vi "register_voltage.vi"(8 "error in (no error)":errorcluster, 11 "DAQVoltage in":refnum<class "DAQVoltage.lvclass">) -> (0 "error out":errorcluster, 3 "DAQVoltage out":refnum<class "DAQVoltage.lvclass">)   [LabVIEW 2025, in "DAQVoltage.lvlib" / "DAQVoltage.lvclass"]
uses:
  DAQVoltage.lvclass
  DAQVoltage.lvclass/DAQVoltage.ctl
  <vilib>/numeric/Random Number (Range) DBL.vi
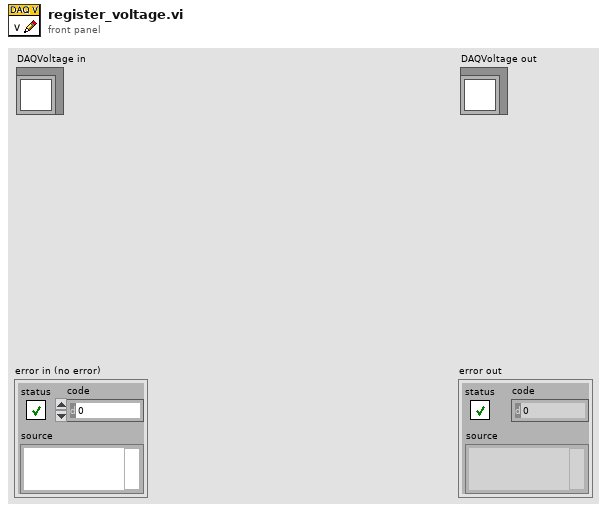
[diagram p1: front panel]
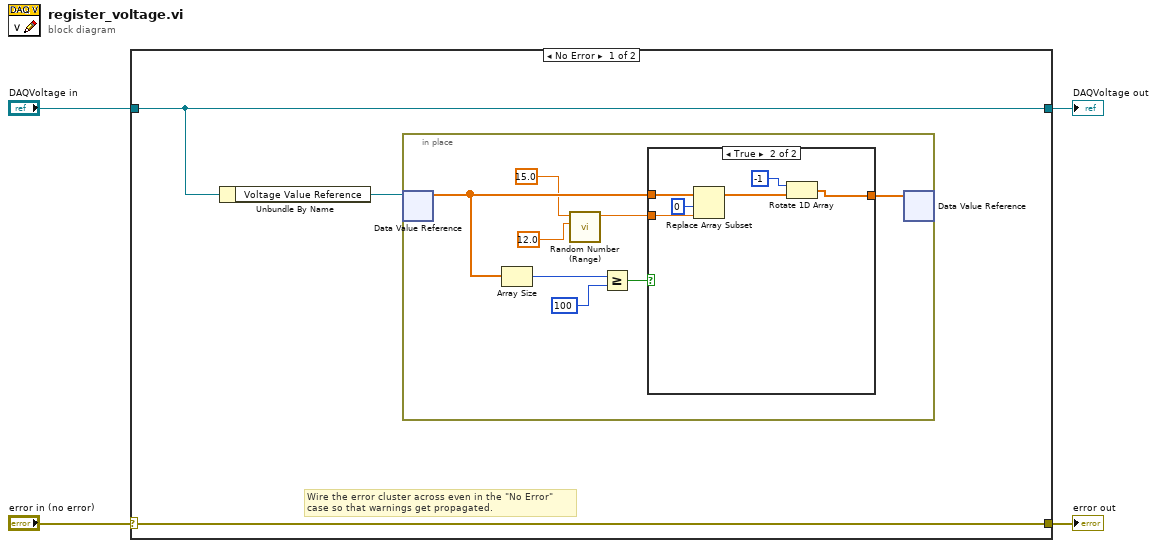
[diagram p0: block diagram]
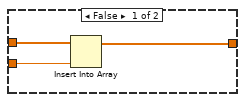
[diagram p2: hidden frame]
diagram:
  n1 = case shown="No Error" "error in (no error)" {
    selector: "error in (no error)" -> [w7 w26]
    tunnel: [w7 w26] -> w3
    tunnel: [w6 w25] -> w1
    tunnel: "DAQVoltage in" -> [w6 w25]
    frame No Error {
      # "Wire the error cluster across even in the \"No Error\"\ncase so that warnings get propagated."
      n2 = Unbundle By Name(w6) -> ("Voltage Value Reference"=w5:refnum<data-value>)
      n3 = in-place {
        n4 = in-place-dvr #1(w5) -> (w13:dbl[])  [unwired: 1 out]
        n5 = Array Size(array=w13) -> (size(s)=w15:i32)
        n6 = call-poly <vilib>:"Random Number (Range).vi"("lower bound (0)"=12.0 ("upper bound (100)"), "upper bound (100)"=15.0) -> ("number"=w8:dbl)  [unwired: 9 in]
        n7 = Greater Or Equal?(x=w15, y=100) -> (x >= y?=w12:bool)
        n8 = case shown="True" w12 {
          tunnel: w13 -> [w18 w24]
          tunnel: [w17 w20] -> w11
          tunnel: w8 -> [w16 w23]
          frame False {
            n9 = Insert Into Array(array=w18, new element=w16) -> (w17:dbl[])  [unwired: 1 in]
          }
          frame True {
            n10 = Replace Array Subset(array=w24, new element=w23, index=0) -> (w21:dbl[])
            n11 = Rotate 1D Array(1:w21, 2:-1 ("n")) -> (0:w20:dbl[])
          }
        }
        n12 = in-place-dvr #1(w11) -> ()  [unwired: 2 out]
      }
    }
    frame Error {
    }
  }
  "error out" <- w3
  "DAQVoltage out" <- w1
